vi "Example_ReadImageFile.vi"() -> ()   [LabVIEW 2020, in "OpenLvVision_Image.lvlib"]
uses:
  OpenLvVision_Image.lvlib
  Management/TypeDef/ImageType.ctl
  Management/Management.lvlib
  File/File.lvlib
panel:
  out "Image":T1(plugin-control)
  in  "Image Path":path
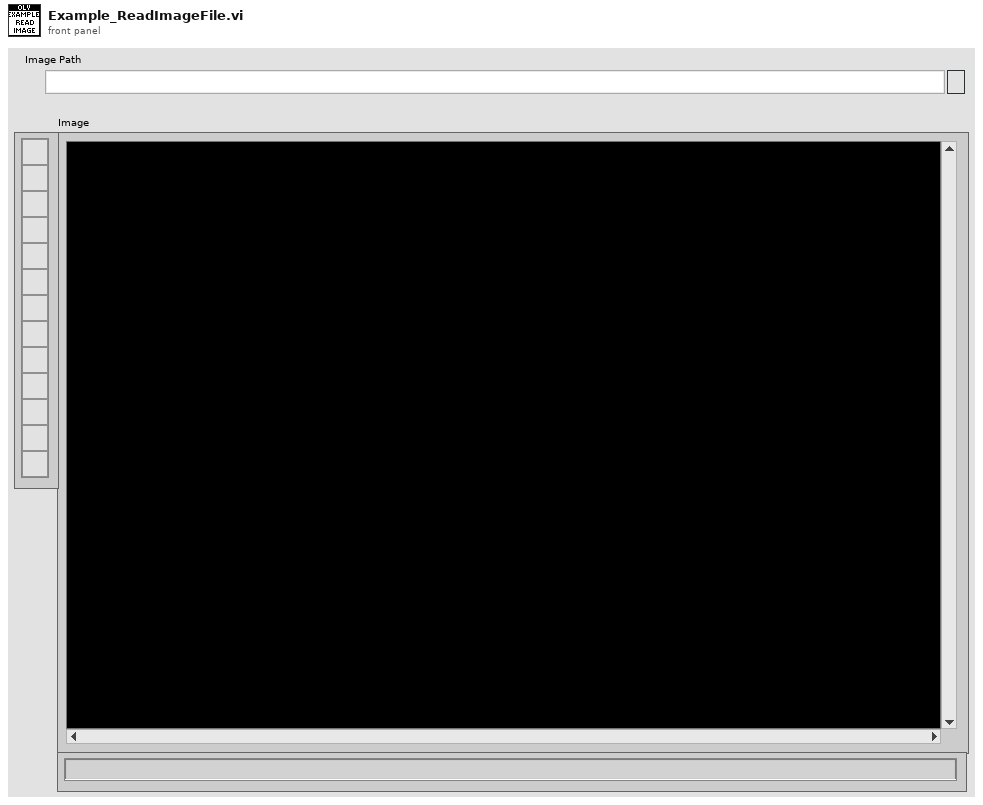
[diagram p1: front panel]
types:
  T1 = typedef "IMAQ Image.ctl" = refnum<image>
  T2 = typedef "OpenLvVision_Image.lvlib/Management.lvlib/ImageType.ctl" = enum16{"Mono U8", "Mono U16", "Mono I16", "Mono SGL", "Color U32", "Color U64"}
  T3 = typedef "OpenLvVision_Image.lvlib/Management.lvlib/Image.ctl" = refnum<image>
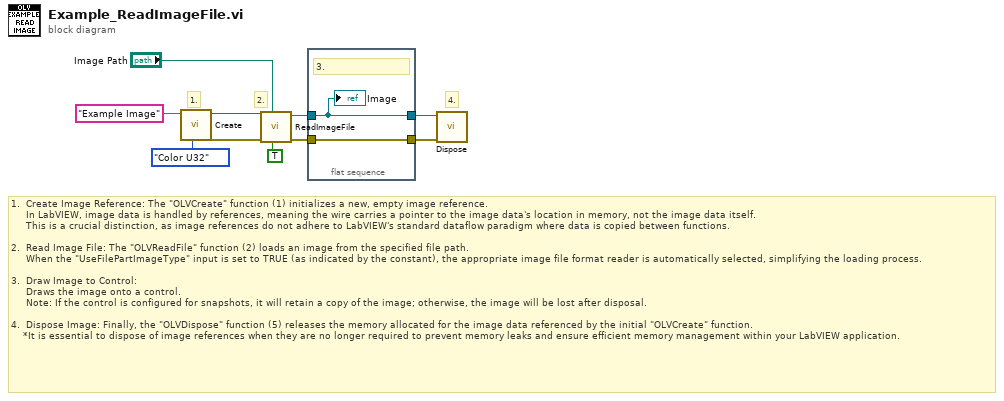
[diagram p0: block diagram]
diagram:
  # "4."
  # "1.  Create Image Reference: The \"OLVCreate\" function (1) initializes a new, empty image reference.\n     In LabVIEW, image data is handled by references, meaning the wire carries a pointer to the image data's location in memory, not the image data itself.\n     This is a crucial distinction, as image references do not adhere to LabVIEW's standard dataflow paradigm where data is copied between functions.\n\n2.  Read Image File: The \"OLVReadFile\" function (2) loads an image from the specified file path.\n     When the \"UseFilePartImageType\" input is set to TRUE (as indicated by the constant), the appropriate image file format reader is automatically selected, simplifying the loading process.\n\n3.  Draw Image to Control:\n     Draws the image onto a control.\n     Note: If the control is configured for snapshots, it will retain a copy of the image; otherwise, the image will be lost after disposal.\n\n4.  Dispose Image: Finally, the \"OLVDispose\" function (5) releases the memory allocated for the image data referenced by the initial \"OLVCreate\" function.\n    *It is essential to dispose of image references when they are no longer required to prevent memory leaks and ensure efficient memory management within your LabVIEW application."
  # "2."
  # "1."
  n1 = call "Create.vi"("Image Type"=ImageType."Color U32", "Image Name"="Example Image") -> ("error out"=w7:errorcluster, "Image Reference Out"=w8:T3)  [unwired: 8 in]
  n2 = call "ReadImageFile.vi"("Use File Path Image Type"=TRUE, "File Path"="Image Path", "error in"=w7, "Image Reference In"=w8) -> ("error out"=w4:errorcluster, "Image Reference Out"=w5:T3)  [unwired: 3 in, 3 out]
  n3 = flat-sequence {
    tunnel: w5 -> [w12]
    tunnel: w4 -> [w11]
    tunnel: [w12] -> w2
    tunnel: [w11] -> w1
    frame #0 {
      # "3."
      "Image" <- w12
    }
  }
  n4 = call "Dispose.vi"("error in"=w1, "Image Reference In"=w2) -> ()  [unwired: 9 in, 1 out]
